vi "Teleop.vi"(10 "Match Info":T1={"Autonomous Elapsed Seconds"=0.0, "TeleOp Elapsed Seconds"=0.0, "Disabled Elapsed Seconds"=0.0, "Visited Autonomous"=FALSE, "Visited TeleOp"=FALSE, "Visited Disabled"=FALSE, "Autonomous Settings"={"Autonomous Style"=enum."Independent", "VI Refnum"=refnum}}, 11 "Call Context":T2) -> ()   [LabVIEW 2013]
doc: "This VI is called for each TeleOp packet received from the DS where the robot is not disabled. It is often used to read from the joysticks and update I/O or to update setpoints for timed control loops. It should complete and return within 20 milliseconds or it may miss DS packets."
uses:
  Robot Global Data.vi
  <vilib>/Rock Robotics/WPI/Solenoid/Deprecated/WPI_SolenoidGetBool.vi
  <vilib>/Rock Robotics/WPI/Solenoid/WPI_SolenoidSetEnum.vi
  <vilib>/Rock Robotics/WPI/Solenoid/WPI_SolenoidValue.ctl
  <vilib>/Rock Robotics/WPI/DriverStation/WPI_DriverStationMatch Info.ctl
  <vilib>/Rock Robotics/WPI/DriverStation/WPI_DriverStationDerivedRobotMode.ctl
panel:
  out "Numeric 1":dbl(slide) scale=0.0..100.0
  out "Boolean 2":bool
  out "Boolean 1":bool
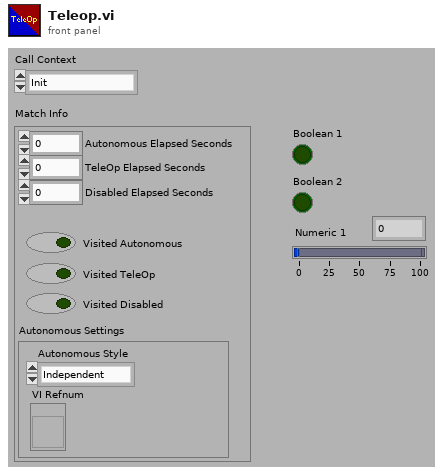
[diagram p1: front panel]
types:
  T1 = typedef "WPI_DriverStationMatch Info.ctl" = cluster{"Autonomous Elapsed Seconds":dbl, "TeleOp Elapsed Seconds":dbl, "Disabled Elapsed Seconds":dbl, "Visited Autonomous":bool, "Visited TeleOp":bool, "Visited Disabled":bool, "Autonomous Settings":cluster{"Autonomous Style":enum16{"Iterative", "Independent"}, "VI Refnum":refnum<vi>}}
  T2 = typedef "WPI_DriverStationDerivedRobotMode.ctl" = enum16{"Init", "Execute", "Stop"}
  T3 = typedef "WPI_RobotDriveDevRef.ctl" = cluster{"DevStatus":errorcluster, "Motors[]":T4[], "Square Inputs":bool, "Max Output":dbl, "Isochronous":bool}
  T4 = typedef "WPI_MotorControlDeviceRef.ctl" = cluster{"DeviceStatus":errorcluster, "Type":enum16{"PWM", "CAN"}, "PWM":cluster{"Digital Module":T5, "PWM Channel":T6, "DeadBand":T7}, "CAN":cluster{"Device Number":u8, "Control Mode":T8, "Semaphore":T9, "Max Vout":dbl}, "Invert":bool, "TransformRef":T10, "InvTransformRef":T10}
  T5 = typedef "FPGA_TypedefDigitalModule.ctl" = enum16{"Digital Module 1", "Digital Module 2"}
  T6 = typedef "FPGA_DIOPWMChannel.ctl" = enum8{"PWM 1", "PWM 2", "PWM 3", "PWM 4", "PWM 5", "PWM 6", "PWM 7", "PWM 8", "PWM 9", "PWM 10", "Invalid"}
  T7 = typedef "WPI_PWMDeadband.ctl" = cluster{"Name":string, "maxPositivePwm":i32, "minPositivePwm":i32, "centerPwm":i32, "maxNegativePwm":i32, "minNegativePwm":i32, "angularRange":u16}
  T8 = typedef "WPI_CANJaguar_ControlMode.ctl" = enum8{"Percent VBus", "Current", "Speed", "Position", "Voltage"}
  T9 = typedef "Semaphore RefNum" = refnum<k1>
  T10 = typedef "WPI_PWMTransform_ConPane.ctl" = refnum<vi>
  T11 = typedef "WPI_JoystickDevRef.ctl" = cluster{"Device":T12}
  T12 = typedef "WPI_JoystickDeviceEnum.ctl" = enum16{"USB 1", "USB 2", "USB 3", "USB 4", "Kinect 1", "Kinect 2"}
  T13 = typedef "WPI_JoystickButtonState.ctl" = cluster{"Button 1":bool, "Button 2":bool, "Button 3":bool, "Button 4":bool, "Button 5":bool, "Button 6":bool, "Button 7":bool, "Button 8":bool, "Button 9":bool, "Button 10":bool, "Button 11":bool, "Button 12":bool}
  T14 = cluster{"axis 1 (x)":dbl, "axis 2 (y)":dbl, "axis 3 (throttle)":dbl, "axis 4":dbl, "axis 5":dbl, "axis 6":dbl}
  T15 = typedef "WPI_AnalogChannelDevRef.ctl" = cluster{"DevStatus":errorcluster, "Analog Module":T16, "Analog Channel":T17}
  T16 = typedef "FPGA_TypedefAnalogModule.ctl" = enum16{"Analog Module 1", "Analog Module 2"}
  T17 = typedef "FPGA_AIChannel.ctl" = enum8{"AI 1", "AI 2", "AI 3", "AI 4", "AI 5", "AI 6", "AI 7", "AI 8", "Invalid"}
  T18 = typedef "WPI_SolenoidDevRef.ctl" = cluster{"DevStatus":errorcluster, "Solenoid Module":T19, "Forward Solenoid Channel":T20, "Reverse Solenoid Channel":T20}
  T19 = typedef "FPGA_TypedefSolenoidModule.ctl" = enum16{"Solenoid Module 1", "Solenoid Module 2"}
  T20 = typedef "WPI_SolenoidChannel.ctl" = enum8{"Solenoid 1", "Solenoid 2", "Solenoid 3", "Solenoid 4", "Solenoid 5", "Solenoid 6", "Solenoid 7", "Solenoid 8", "Invalid"}
  T21 = typedef "WPI_SolenoidValue.ctl" = enum16{"Off", "On", "Forward", "Reverse"}
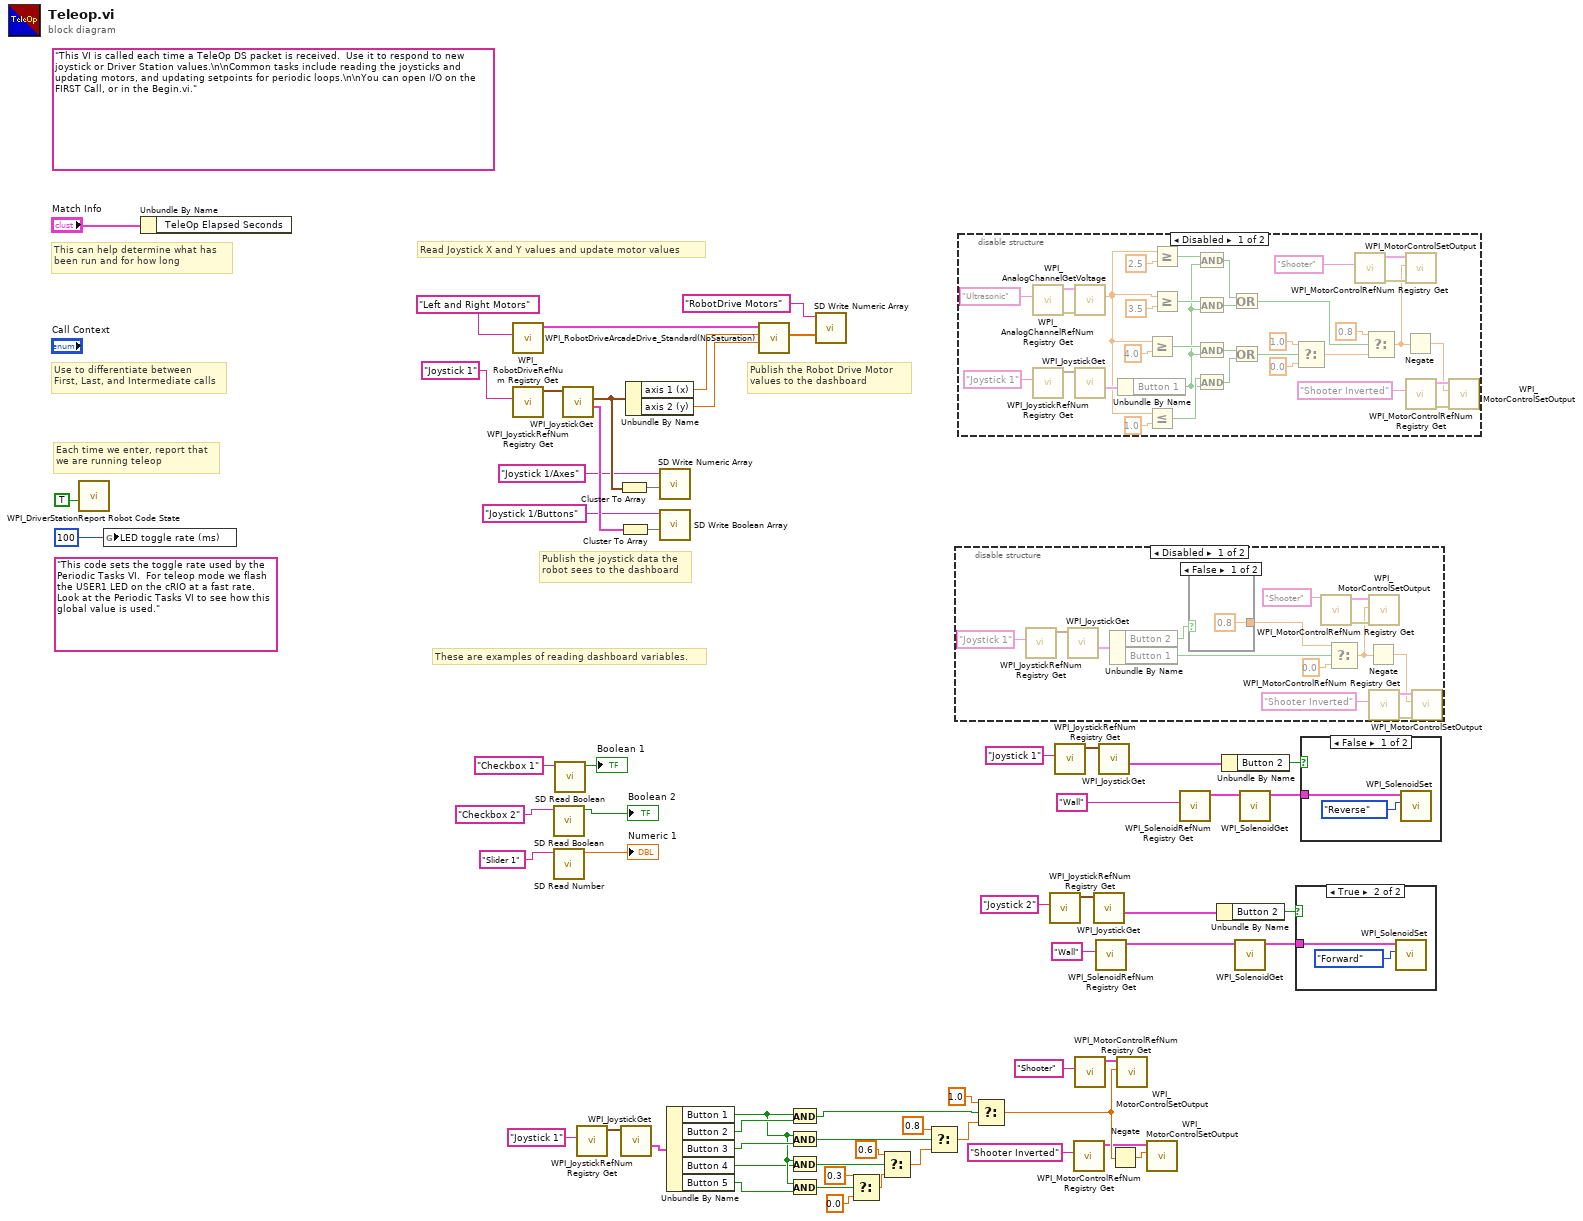
[diagram p0: block diagram]
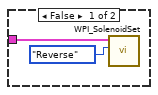
[diagram p2: hidden frame]
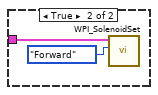
[diagram p3: hidden frame]
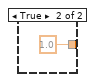
[diagram p5: hidden frame]
diagram:
  (unwired) "This code sets the toggle rate used by the Periodic Tasks VI.  For teleop mode we flash the USER1 LED on the cRIO at a fast rate.  Look at the Periodic Tasks VI to see how this global value is used."
  (unwired) "This VI is called each time a TeleOp DS packet is received.  Use it to respond to new joystick or Driver Station values.\n\nCommon tasks include reading the joysticks and updating motors, and updating setpoints for periodic loops.\n\nYou can open I/O on the FIRST Call, or in the Begin.vi."
  # "These are examples of reading dashboard variables."
  # "Publish the Robot Drive Motor\nvalues to the dashboard"
  # "Publish the joystick data the\nrobot sees to the dashboard"
  # "Each time we enter, report that\nwe are running teleop"
  # "Use to differentiate between\nFirst, Last, and Intermediate calls"
  # "This can help determine what has\nbeen run and for how long"
  # "Read Joystick X and Y values and update motor values"
  n1 = call <vilib>:"WPI_DriverStationReport Robot Code State.vi"("TeleOp"=TRUE ("Autonomous")) -> ()  [unwired: 10 in, 1 out]
  n2 = global write "Robot Global Data.vi" "LED toggle rate (ms)"(u32 100 ("LED ms toggle rate")) -> ()
  n3 = Unbundle By Name("Match Info") -> ()  [unwired: 1 out]
  n4 = call <vilib>:"WPI_RobotDriveRefNum Registry Get.vi"("refnum name"="Left and Right Motors") -> ("RobotDriveDevRef"=w61:T3)  [unwired: 1 in, 9 out]
  n5 = call <vilib>:"WPI_JoystickRefNum Registry Get.vi"("refnum name"="Joystick 1") -> ("JoystickDevRef"=w57:T11)  [unwired: 1 in, 9 out]
  n6 = call <vilib>:"SD Read Boolean.vi"("Name"="Checkbox 2" ("refnum name")) -> ("Boolean"=→"Boolean 2":bool)  [unwired: 8 in, 2 out]
  n7 = call <vilib>:"SD Read Number.vi"("Name"="Slider 1" ("refnum name")) -> ("Numeric"=→"Numeric 1":dbl)  [unwired: 8 in, 2 out]
  n8 = call <vilib>:"SD Read Boolean.vi"("Name"="Checkbox 1" ("refnum name")) -> ("Boolean"=→"Boolean 1":bool)  [unwired: 8 in, 2 out]
  n9 = call <vilib>:"WPI_JoystickGet.vi"("JoystickDevRef"=w57) -> ("Buttons"=w54:T13, "Axes"=w51:T14)  [unwired: 1 in, 4 out]
  n10 = call <vilib>:"WPI_JoystickRefNum Registry Get.vi"("refnum name"="Joystick 1") -> ("JoystickDevRef"=w24:T11)  [unwired: 9 in, 1 out]
  n11 = Cluster To Array(cluster=w51) -> (array=w50:dbl[])
  n12 = Cluster To Array(cluster=w54) -> (array=w53:bool[])
  n13 = call <vilib>:"WPI_JoystickGet.vi"("JoystickDevRef"=w24) -> ("Buttons"=w26:T13)  [unwired: 4 in, 2 out]
  n14 = Unbundle By Name(w51) -> ("axis 1 (x)"=w60:dbl, "axis 2 (y)"=w59:dbl)
  n15 = call <vilib>:"SD Write Numeric Array.vi"("Numeric Array"=w50, "Name"="Joystick 1/Axes") -> ()  [unwired: 8 in, 2 out]
  n16 = call <vilib>:"SD Write Boolean Array.vi"("Boolean Array"=w53, "Name"="Joystick 1/Buttons") -> ()  [unwired: 8 in, 2 out]
  n17 = Unbundle By Name(w26) -> ("Button 1"=w21:bool, "Button 2"=w23:bool, "Button 3"=w22:bool, "Button 4"=w20:bool, "Button 5"=w19:bool)
  n18 = call <vilib>:"WPI_RobotDriveArcadeDrive_Standard(NoSaturation).vi"("Y axis value"=w59, "X axis value"=w60, "RobotDriveDevRef"=w61) -> ("Motor Values"=w47:dbl[])  [unwired: 1 in, 7 out]
  n19 = And(x=w21, y=w23) -> (x .and. y?=w18:bool)
  n20 = And(x=w21, y=w22) -> (x .and. y?=w12:bool)
  n21 = And(x=w21, y=w20) -> (x .and. y?=w13:bool)
  n22 = And(x=w21, y=w19) -> (x .and. y?=w14:bool)
  n23 = call <vilib>:"SD Write Numeric Array.vi"("Numeric Array"=w47, "Name"="RobotDrive Motors") -> ()  [unwired: 8 in, 2 out]
  n24 = Select(t=0.3, s=w14, f=0.0) -> (s? t:f=w15:dbl)
  n25 = Select(t=0.6, s=w13, f=w15) -> (s? t:f=w16:dbl)
  n26 = Select(t=0.8, s=w12, f=w16) -> (s? t:f=w17:dbl)
  n27 = disable-structure shown="Disabled" {
    frame Disabled {
      n28 = call <vilib>:"WPI_JoystickRefNum Registry Get.vi"("refnum name"="Joystick 1") -> ("JoystickDevRef"=w77:T11)  [unwired: 9 in, 1 out]
      n29 = call <vilib>:"WPI_JoystickGet.vi"("JoystickDevRef"=w77) -> ("Buttons"=w76:T13)  [unwired: 4 in, 2 out]
      n30 = Unbundle By Name(w76) -> ("Button 2"=w75:bool, "Button 1"=w74:bool)
      n31 = case shown="False" w75 {
        tunnel: [0.8 1.0] -> w73
        frame False {
        }
        frame True {
        }
      }
      n32 = call <vilib>:"WPI_MotorControlRefNum Registry Get.vi"("refnum name"="Shooter") -> ("error out"=w70:errorcluster, "MotorControlDevRef"=w71:T4)  [unwired: 9 in]
      n33 = Select(t=w73, s=w74, f=0.0) -> (s? t:f=w65:dbl)
      n34 = Negate(x=w65) -> (-x=w64:dbl)
      n35 = call <vilib>:"WPI_MotorControlSetOutput.vi"("error in (no error)"=w70, "Output"=w65, "MotorControlDevRef"=w71) -> ()  [unwired: 6 in, 3 out]
      n36 = call <vilib>:"WPI_MotorControlRefNum Registry Get.vi"("refnum name"="Shooter Inverted") -> ("error out"=w67:errorcluster, "MotorControlDevRef"=w68:T4)  [unwired: 9 in]
      n37 = call <vilib>:"WPI_MotorControlSetOutput.vi"("error in (no error)"=w67, "Output"=w64, "MotorControlDevRef"=w68) -> ()  [unwired: 6 in, 3 out]
    }
    frame Disabled {
    }
  }
  n38 = disable-structure shown="Disabled" {
    frame Disabled {
      n39 = call <vilib>:"WPI_AnalogChannelRefNum Registry Get.vi"("refnum name"="Ultrasonic") -> ("error out"=w110:errorcluster, "AIDeviceRef"=w109:T15)  [unwired: 9 in]
      n40 = call <vilib>:"WPI_JoystickRefNum Registry Get.vi"("refnum name"="Joystick 1") -> ("JoystickDevRef"=w113:T11)  [unwired: 9 in, 1 out]
      n41 = call <vilib>:"WPI_AnalogChannelGetVoltage.vi"("error in (no error)"=w110, "AIDeviceRef"=w109) -> ("Voltage"=w97:dbl)  [unwired: 7 in, 2 out]
      n42 = call <vilib>:"WPI_JoystickGet.vi"("JoystickDevRef"=w113) -> ("Buttons"=w112:T13)  [unwired: 4 in, 2 out]
      n43 = Unbundle By Name(w112) -> ("Button 1"=w94:bool)
      n44 = Greater Or Equal?(x=w97, y=4.0) -> (x >= y?=w95:bool)
      n45 = Less Or Equal?(x=w97, y=1.0) -> (x <= y?=w99:bool)
      n46 = Greater Or Equal?(x=w97, y=2.5) -> (x >= y?=w102:bool)
      n47 = Greater Or Equal?(x=w97, y=3.5) -> (x >= y?=w107:bool)
      n48 = And(x=w102, y=w94) -> (x .and. y?=w101:bool)
      n49 = And(x=w107, y=w94) -> (x .and. y?=w105:bool)
      n50 = And(x=w95, y=w94) -> (x .and. y?=w93:bool)
      n51 = And(x=w99, y=w94) -> (x .and. y?=w98:bool)
      n52 = Or(x=w101, y=w105) -> (x .or. y?=w104:bool)
      n53 = Or(x=w93, y=w98) -> (x .or. y?=w92:bool)
      n54 = Select(t=1.0, s=w92, f=0.0) -> (s? t:f=w89:dbl)
      n55 = call <vilib>:"WPI_MotorControlRefNum Registry Get.vi"("refnum name"="Shooter") -> ("error out"=w84:errorcluster, "MotorControlDevRef"=w83:T4)  [unwired: 9 in]
      n56 = Select(t=0.8, s=w104, f=w89) -> (s? t:f=w82:dbl)
      n57 = Negate(x=w82) -> (-x=w81:dbl)
      n58 = call <vilib>:"WPI_MotorControlSetOutput.vi"("error in (no error)"=w84, "Output"=w82, "MotorControlDevRef"=w83) -> ()  [unwired: 6 in, 3 out]
      n59 = call <vilib>:"WPI_MotorControlRefNum Registry Get.vi"("refnum name"="Shooter Inverted") -> ("error out"=w86:errorcluster, "MotorControlDevRef"=w85:T4)  [unwired: 9 in]
      n60 = call <vilib>:"WPI_MotorControlSetOutput.vi"("error in (no error)"=w86, "Output"=w81, "MotorControlDevRef"=w85) -> ()  [unwired: 6 in, 3 out]
    }
    frame Enabled {
    }
  }
  n61 = Select(t=1.0, s=w18, f=w17) -> (s? t:f=w3:dbl)
  n62 = call <vilib>:"WPI_JoystickRefNum Registry Get.vi"("refnum name"="Joystick 2") -> ("JoystickDevRef"=w29:T11)  [unwired: 9 in, 1 out]
  n63 = call <vilib>:"WPI_JoystickRefNum Registry Get.vi"("refnum name"="Joystick 1") -> ("JoystickDevRef"=w38:T11)  [unwired: 9 in, 1 out]
  n64 = call <vilib>:"WPI_MotorControlRefNum Registry Get.vi"("refnum name"="Shooter Inverted") -> ("MotorControlDevRef"=w2:T4)  [unwired: 9 in, 1 out]
  n65 = call <vilib>:"WPI_MotorControlRefNum Registry Get.vi"("refnum name"="Shooter") -> ("MotorControlDevRef"=w5:T4)  [unwired: 9 in, 1 out]
  n66 = call <vilib>:"WPI_JoystickGet.vi"("JoystickDevRef"=w29) -> ("Buttons"=w31:T13)  [unwired: 4 in, 2 out]
  n67 = call <vilib>:"WPI_SolenoidRefNum Registry Get.vi"("refnum name"="Wall") -> ("SolenoidDevRef"=w28:T18)  [unwired: 9 in, 1 out]
  n68 = call <vilib>:"WPI_JoystickGet.vi"("JoystickDevRef"=w38) -> ("Buttons"=w36:T13)  [unwired: 4 in, 2 out]
  n69 = Negate(x=w3) -> (-x=w4:dbl)
  n70 = call <vilib>:"WPI_MotorControlSetOutput.vi"("Output"=w3, "MotorControlDevRef"=w5) -> ()  [unwired: 7 in, 3 out]
  n71 = call <vilib>:"WPI_MotorControlSetOutput.vi"("Output"=w4, "MotorControlDevRef"=w2) -> ()  [unwired: 7 in, 3 out]
  n72 = call <vilib>:"WPI_SolenoidRefNum Registry Get.vi"("refnum name"="Wall") -> ("SolenoidDevRef"=w39:T18)  [unwired: 9 in, 1 out]
  n73 = Unbundle By Name(w31) -> ("Button 2"=w32:bool)
  n74 = Unbundle By Name(w36) -> ("Button 2"=w35:bool)
  n75 = call-poly <vilib>:"WPI_SolenoidGet.vi"("SolenoidDevRef"=w28) -> ("SolenoidDevRef"=w33:T18)  [unwired: 8 in, 2 out]
  n76 = call-poly <vilib>:"WPI_SolenoidGet.vi"("SolenoidDevRef"=w39) -> ("SolenoidDevRef"=w34:T18)  [unwired: 8 in, 2 out]
  n77 = case shown="True" w32 {
    tunnel: w33 -> [w116 w118]
    frame False {
      n78 = call-poly <vilib>:"WPI_SolenoidSet.vi"("Value"=WPI_SolenoidValue."Reverse", "SolenoidDevRef"=w116) -> ()  [unwired: 8 in, 2 out]
    }
    frame True {
      n79 = call-poly <vilib>:"WPI_SolenoidSet.vi"("Value"=WPI_SolenoidValue."Forward", "SolenoidDevRef"=w118) -> ()  [unwired: 8 in, 2 out]
    }
  }
  n80 = case shown="False" w35 {
    tunnel: w34 -> [w120 w122]
    frame False {
      n81 = call-poly <vilib>:"WPI_SolenoidSet.vi"("Value"=WPI_SolenoidValue."Reverse", "SolenoidDevRef"=w120) -> ()  [unwired: 8 in, 2 out]
    }
    frame True {
      n82 = call-poly <vilib>:"WPI_SolenoidSet.vi"("Value"=WPI_SolenoidValue."Forward", "SolenoidDevRef"=w122) -> ()  [unwired: 8 in, 2 out]
    }
  }
